vi "Add Task.vi"(8 "error in (no error)":errorcluster, 10 "Task":refnum<class>, 11 "Work Dispatcher in":refnum<class "Work Dispatcher.lvclass">) -> (0 "error out":errorcluster, 3 "Work Dispatcher out":refnum<class "Work Dispatcher.lvclass">)   [LabVIEW 2023, in "Work Dispatcher.lvlib" / "Work Dispatcher.lvclass"]
doc: "Add a task to the pending work queue."
uses:
  Work Dispatcher.lvclass
  c:/dev/_r/4/eng/lv-core/lvpostprocessingd/lv_mc_x86_64/dist_i386/vi.lib/ActorFramework/Actor/Actor.lvclass
  <vilib>/ActorFramework/Actor/Actor.lvclass/Actor.ctl
  <vilib>/ActorFramework/Message Enqueuer/Message Enqueuer.lvclass/Message Enqueuer.ctl
  Work Dispatcher.lvclass/Work Dispatcher.ctl
  Person Messages/Process Job Msg/Process Job Msg.lvclass/Process Job Msg.ctl
  Work Dispatcher Messages/Add Task Msg/Add Task Msg.lvclass/Add Task Msg.ctl
  <vilib>/ActorFramework/Message Enqueuer/Init from Existing Queue.vi
  <vilib>/ActorFramework/Message Enqueuer/Enqueue.vi
  Person Messages/Process Job Msg/Process Job Msg.lvclass
  c:/dev/_r/4/eng/lv-core/lvpostprocessingd/lv_mc_x86_64/dist_i386/vi.lib/ActorFramework/Message/Message.lvclass
  Work Dispatcher Messages/Add Task Msg/Add Task Msg.lvclass
  <vilib>/ActorFramework/Message Priority Queue/Priority Enqueue.vi
  <vilib>/ActorFramework/Message Enqueuer/Message Enqueuer.lvclass
  <vilib>/ActorFramework/Actor/Actor.lvclass
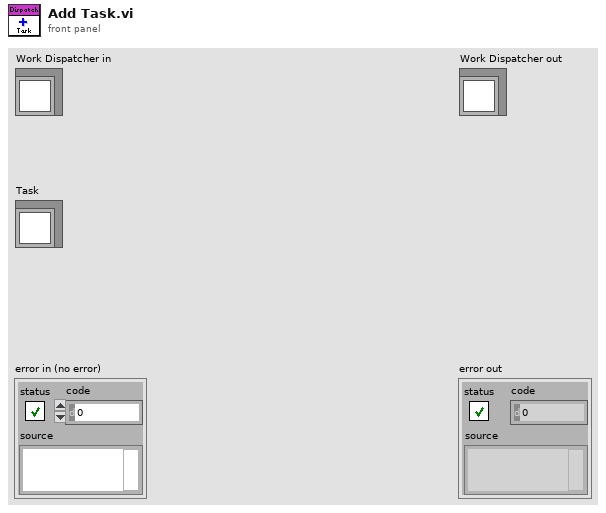
[diagram p1: front panel]
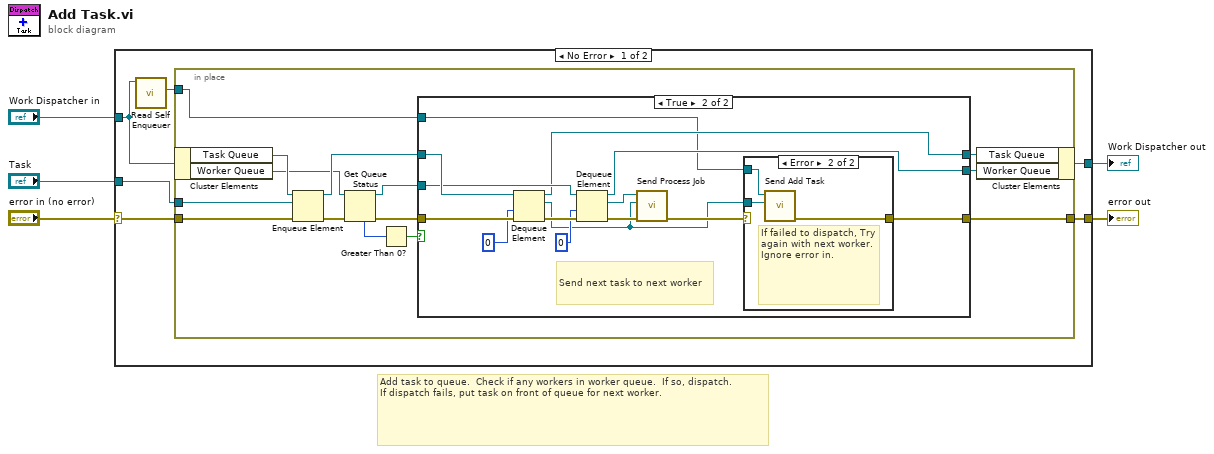
[diagram p0: block diagram]
diagram:
  # "Add task to queue.  Check if any workers in worker queue.  If so, dispatch.\nIf dispatch fails, put task on front of queue for next worker."
  n1 = case shown="No Error" "error in (no error)" {
    selector: "error in (no error)" -> [w9 w48]
    tunnel: [w10 w48] -> w4
    tunnel: [w11 w47] -> w2
    tunnel: "Work Dispatcher in" -> [w7 w47]
    tunnel: "Task" -> [w8 _]
    frame No Error {
      n2 = call <vilib>:"Read Self Enqueuer.vi"("Actor"=w7) -> ("Self Enqueuer"=w6:refnum<class "Message Enqueuer.lvclass">)  [unwired: 10 in]
      n3 = in-place "In Place Element Structure" {
        in-place-border: [w23] -> w10
        in-place-border: w9 -> [w22]
        in-place-border: w8 -> [w20]
        in-place-border: w6 -> [w12]
        n4 = in-place-cluster #1 ("Unbundle / Bundle Elements")(w7) -> ("Task Queue"=w21:refnum<queue>, "Worker Queue"=w18:refnum<queue>)
        n5 = Enqueue Element(queue=w21, element=w20, error in (no error)=w22) -> (queue out=w19:refnum<queue>, error out=w17:errorcluster)  [unwired: 1 in, 1 out]
        n6 = Get Queue Status(queue=w18, error in (no error)=w17) -> (queue out=w13:refnum<queue>, error out=w14:errorcluster, # elements in queue=w16:i32)  [unwired: 1 in, 5 out]
        n7 = Greater Than 0?(x=w16) -> (x > 0?=w15:bool)
        n8 = case shown="True" w15 {
          tunnel: w19 -> [w28 w42]
          tunnel: w13 -> [w26 w41]
          tunnel: w14 -> [w27 w39]
          tunnel: [w27 w32] -> w23
          tunnel: [w26 w38] -> w24
          tunnel: [w28 w37] -> w25
          tunnel: w12 -> [_ w29]
          frame False {
          }
          frame True {
            # "Send next task to next worker"
            n9 = Dequeue Element(queue=w42, timeout in ms (-1)=0, error in (no error)=w39) -> (queue out=w37:refnum<queue>, element=w30:refnum<class>, error out=w40:errorcluster)  [unwired: 1 out]
            n10 = Dequeue Element(queue=w41, timeout in ms (-1)=0, error in (no error)=w40) -> (queue out=w38:refnum<queue>, element=w35:refnum<class "Message Enqueuer.lvclass">, error out=w36:errorcluster)  [unwired: 1 out]
            n11 = call "Send Process Job.vi"("error in (no error)"=w36, "Task"=w30, "Message Enqueuer"=w35) -> ("error out"=w31:errorcluster)  [unwired: 7 in, 1 out]
            n12 = case shown="Error" w31 {
              selector: w31 -> [w43 _]
              tunnel: w30 -> [_ w45]
              tunnel: [w43 w46] -> w32
              tunnel: w29 -> [_ w44]
              frame No Error {
              }
              frame Error {
                # "If failed to dispatch, Try again with next worker.  Ignore error in."
                n13 = call "Send Add Task.vi"("Task"=w45, "Message Enqueuer"=w44) -> ("error out"=w46:errorcluster)  [unwired: 8 in, 1 out]
              }
            }
          }
        }
        n14 = in-place-cluster #1 ("Unbundle / Bundle Elements")("Task Queue"=w25, "Worker Queue"=w24) -> (w11:refnum<class "Work Dispatcher.lvclass">)
      }
    }
    frame Error {
    }
  }
  "error out" <- w4
  "Work Dispatcher out" <- w2
